vi "Check Response&Variables Correspondence.vi"(7 "Command/Response Refnum in":T1 format="%.0x", 8 "error in (no error)":errorcluster, 9 "Variables in":string[](array[string]), 11 "Linked Channels in":cluster{"Variable Name":string, "GUID":string}[](array[cluster])) -> (0 "error out":errorcluster, 3 "Linked Channels out":T2[](array[typedef]))   [LabVIEW 2018, in "Instrument Addon Scripting API.lvlib"]
uses:
  Instrument Addon Scripting API.lvlib
  Addon/Addon Shared/Types/Linked Channel Cluster.ctl
  <vilib>/NI Veristand/Custom Device API/Custom Device Item Ref.ctl
  Addon/Addon Shared/SubVIs/Constants.vi
  Addon/Addon Shared/Instrument Addon Shared.lvlib
  <vilib>/NI VeriStand/Custom Device API/Custom Device API.lvlib
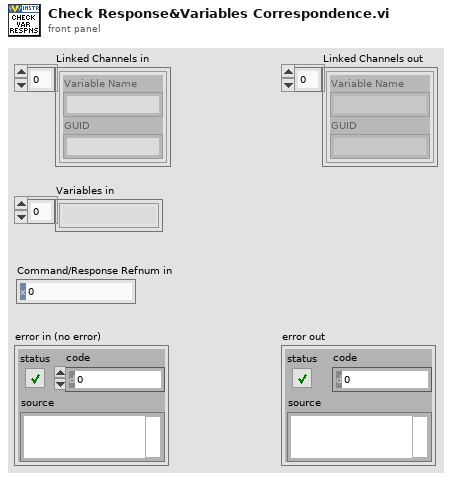
[diagram p1: front panel]
types:
  T1 = typedef "Custom Device API.lvlib/Custom Device Item Ref.ctl" = u64
  T2 = typedef "Instrument Addon Shared.lvlib/Linked Channel Cluster.ctl" = cluster{"Variable Name":string, "GUID":string}
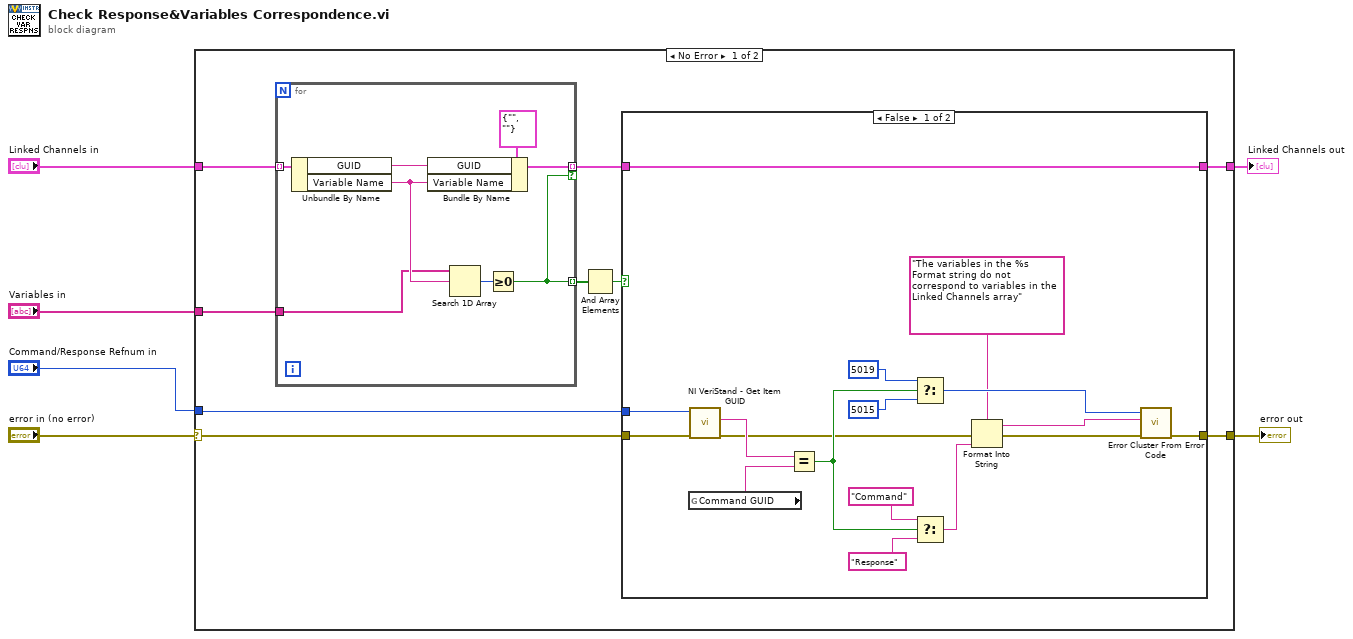
[diagram p0: block diagram]
diagram:
  n1 = case shown="No Error" "error in (no error)" {
    selector: "error in (no error)" -> [w8 w43]
    tunnel: "Linked Channels in" -> [w15 w44]
    tunnel: [w12 w43] -> w2
    tunnel: [w10 w44] -> w3
    tunnel: "Variables in" -> [w9 _]
    tunnel: "Command/Response Refnum in" -> [w7 _]
    frame No Error {
      n2 = for {
        tunnel: w15 -> [w41] mode=indexing
        tunnel: [w39] -> w11 mode=indexing if=w36
        tunnel: [w36] -> w14 mode=indexing
        tunnel: w9 -> [w35]
        n3 = Unbundle By Name(w41) -> ("GUID"=w40:string, "Variable Name"=w37:string)
        n4 = Bundle By Name(cluster=T2 {"Variable Name"="", "GUID"=""} ("Linked Channel"), "GUID"=w40, "Variable Name"=w37) -> (w39:T2)
        n5 = Search 1D Array(1D array=w35, element=w37) -> (index of element=w38:i32)  [unwired: 1 in]
        n6 = Greater Or Equal To 0?(x=w38) -> (x >= 0?=w36:bool)
      }
      n7 = And Array Elements(Boolean array=w14) -> (logical AND=w13:bool)
      n8 = case shown="False" w13 {
        tunnel: [w32 w33] -> w12
        tunnel: w11 -> [w31 w34]
        tunnel: [w31 w34] -> w10
        tunnel: w8 -> [w20 w33]
        tunnel: w7 -> [w19 _]
        frame False {
          n9 = global read "Constants.vi" "Command GUID"() -> (w29:string)
          n10 = call <vilib>:"NI VeriStand - Get Item GUID.vi"("error in (no error)"=w20, "Item Ref in"=w19) -> ("error out"=w27:errorcluster, "GUID"=w28:string)  [unwired: 7 in, 1 out]
          n11 = Equal?(x=w28, y=w29) -> (x = y?=w30:bool)
          n12 = Select(t=5019 ("error code (0)"), s=w30, f=5015 ("error code (0)")) -> (s? t:f=w18:i32)
          n13 = Select(t="Command", s=w30, f="Response") -> (s? t:f=w26:string)
          n14 = Format Into String(format string="The variables in the %s Format string do not correspond to variables in the Linked Channels array" ("error message (\"\")"), error in=w27, w26) -> (resulting string=w16:string, error out=w21:errorcluster)  [unwired: 1 in]
          n15 = call <vilib>:"Error Cluster From Error Code.vi"("error in (no error)"=w21, "error message (\"\")"=w16, "error code (0)"=w18) -> ("error out"=w32:errorcluster)  [unwired: 6 in]
        }
        frame True {
        }
      }
    }
    frame Error {
    }
  }
  "Linked Channels out" <- w3
  "error out" <- w2
